vi "Pose3d_ToPose2d.vi"(11 "in Pose3d":T4={"Translation3d"={"X"=0.0, "Y"=0.0, "Z"=0.0}, "Rotation3d"={"Q_quaternion"={"R"=1.0, "V"=[0.0, 0.0, 0.0]}}} {"Translation3d"."Z" format="%14.3f"; "Translation3d"."Y" format="%14.3f"; "Translation3d"."X" format="%14.3f"}) -> (3 "out Pose2d":T1={"TRANSLATION"={"X"=0.0, "Y"=0.0}, "ROTATION"={"VALUE"=0.0, "COS"=1.0, "SIN"=0.0}} {"ROTATION"."SIN" format="%13.4f"; "ROTATION"."COS" format="%13.4f"; "ROTATION"."VALUE" format="%13.4f"; "TRANSLATION"."Y" format="%14.3f"; "TRANSLATION"."X" format="%14.3f"})   [LabVIEW 2019, in "Trajectory_Library.lvlib"]
doc: "Returns a Pose2d representing this Pose3d projected into the X-Y plane.\n\nParameter:\n - IN POSE3D - Current POSE data structure\n\nReturns:\n - out POSE2D - A Pose2d representing this Pose3d projected into the X-Y plane."
uses:
  Trajectory_Library.lvlib
  TypeDef/TRANSLATION3D.ctl
  TypeDef/QUATERNION.ctl
  TypeDef/ROTATION3D.ctl
  TypeDef/POSE3D.ctl
  TypeDef/TRANSLATION2D.ctl
  TypeDef/ROTATION2D.ctl
  TypeDef/POSE2D.ctl
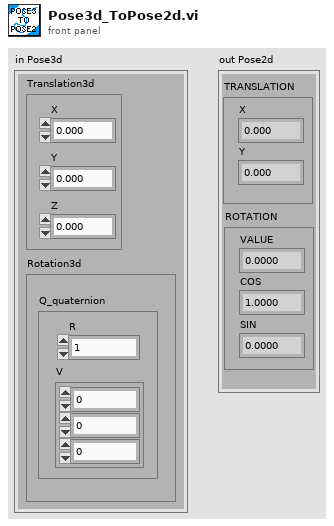
[diagram p1: front panel]
types:
  T1 = typedef "Trajectory_Library.lvlib/POSE2D.ctl" = cluster{"TRANSLATION":T2, "ROTATION":T3}
  T2 = typedef "Trajectory_Library.lvlib/TRANSLATION2D.ctl" = cluster{"X":dbl, "Y":dbl}
  T3 = typedef "Trajectory_Library.lvlib/ROTATION2D.ctl" = cluster{"VALUE":dbl, "COS":dbl, "SIN":dbl}
  T4 = typedef "Trajectory_Library.lvlib/POSE3D.ctl" = cluster{"Translation3d":T5, "Rotation3d":T6}
  T5 = typedef "Trajectory_Library.lvlib/TRANSLATION3D.ctl" = cluster{"X":dbl, "Y":dbl, "Z":dbl}
  T6 = typedef "Trajectory_Library.lvlib/ROTATION3D.ctl" = cluster{"Q_quaternion":T7}
  T7 = typedef "Trajectory_Library.lvlib/QUATERNION.ctl" = cluster{"R":dbl, "V":dbl[]}
  T8 = typedef "WPILib_Math.lvlib/ROTATION3D.ctl" = cluster{"Q_quaternion":T9}
  T9 = typedef "WPILib_Math.lvlib/QUATERNION.ctl" = cluster{"R":dbl, "V":dbl[]}
  T10 = typedef "WPILib_Math.lvlib/TRANSLATION3D.ctl" = cluster{"X":dbl, "Y":dbl, "Z":dbl}
  T11 = typedef "WPILib_Math.lvlib/TRANSLATION2D.ctl" = cluster{"X":dbl, "Y":dbl}
  T12 = typedef "WPILib_Math.lvlib/ROTATION2D.ctl" = cluster{"VALUE":dbl, "COS":dbl, "SIN":dbl}
  T13 = typedef "WPILib_Math.lvlib/POSE2D.ctl" = cluster{"TRANSLATION":T11, "ROTATION":T12}
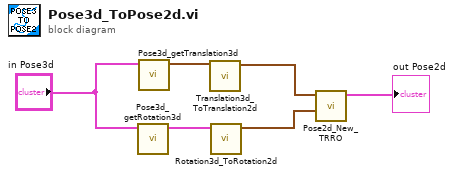
[diagram p0: block diagram]
diagram:
  n1 = call "Pose3d_getRotation3d.vi"("in Pose3d"="in Pose3d") -> ("out Rotation3d"=w4:T8)  [unwired: 10 in]
  n2 = call "Pose3d_getTranslation3d.vi"("in Pose3d"="in Pose3d") -> ("out Translation3d"=w5:T10)  [unwired: 10 in]
  n3 = call "Translation3d_ToTranslation2d.vi"("In Translation3d"=w5) -> ("Translation2d"=w3:T11)  [unwired: 10 in]
  n4 = call "Rotation3d_ToRotation2d.vi"("in Rotation3d"=w4) -> ("out Rotation2d"=w2:T12)  [unwired: 10 in]
  n5 = call "Pose2d_New_TRRO.vi"("ROTATION"=w2, "TRANSLATION"=w3) -> ("outPOSE"=→"out Pose2d":T13)  [unwired: 9 in]
